vi "InsertIntoArray.vi"(6 "input array":dbl[](array[numeric]), 9 "new element 1":dbl, 10 "new element 0":dbl) -> (3 "output array":dbl[](array[numeric]))   [LabVIEW 2014]
panel:
  # "This one only works for doubles"
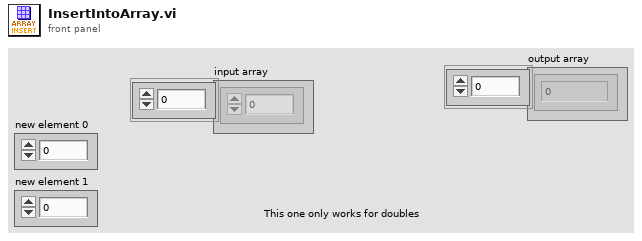
[diagram p1: front panel]
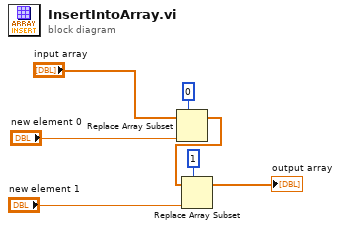
[diagram p0: block diagram]
diagram:
  n1 = Replace Array Subset(array="input array", new element="new element 0", index=0) -> (w5:dbl[])
  n2 = Replace Array Subset(array=w5, new element="new element 1", index=1) -> (→"output array":dbl[])
